vi "timeout.vi"(0 "Limit In":i32, 11 "Strat Time In":i32) -> (4 "Timeout?":bool, 15 "Strat Time Out":i32)   [LabVIEW 2014]
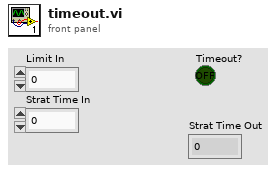
[diagram p1: front panel]
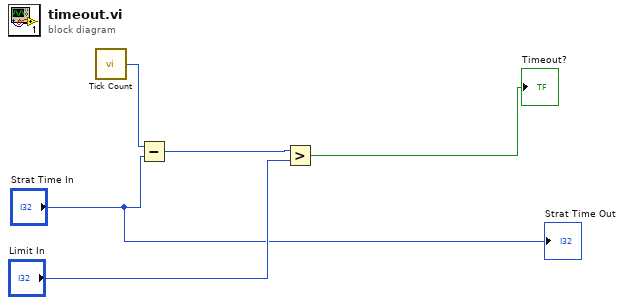
[diagram p0: block diagram]
diagram:
  n1 = call "Tick Count"() -> ("Tick Count(Ticks)"=w1:u32)
  n2 = Subtract(x=w1, y="Strat Time In") -> (x-y=w2:u32)
  n3 = Greater?(x=w2, y="Limit In") -> (0:→"Timeout?":bool)
  "Strat Time Out" <- "Strat Time In"
